vi "Model - DeInit.vi"(8 "error in (no error)":errorcluster, 11 "View Model":T1) -> (0 "error out":errorcluster)   [LabVIEW 2017]
doc: "De-Initialize all View Model Components."
uses:
  Controls/View Model.ctl
  Controls/Shared Model.ctl
  Error Handler/Controls/Error Model.ctl
  Error Handler/Controls/Error Data.ctl
  Error Handler/Controls/Error Type.ctl
  Error Handler/Controls/Error Source.ctl
  Configuration/Controls/Config Model.ctl
  Configuration/Controls/Config CMD.ctl
  Configuration/Controls/Config Command.ctl
  Controller/Controls/Controller Model.ctl
  Controller/Controls/Controller Overhead.ctl
  Controller/Controls/Controller Transaction.ctl
  Controller/Controls/Controller State.ctl
  Configuration/Controls/Config Data Record.ctl
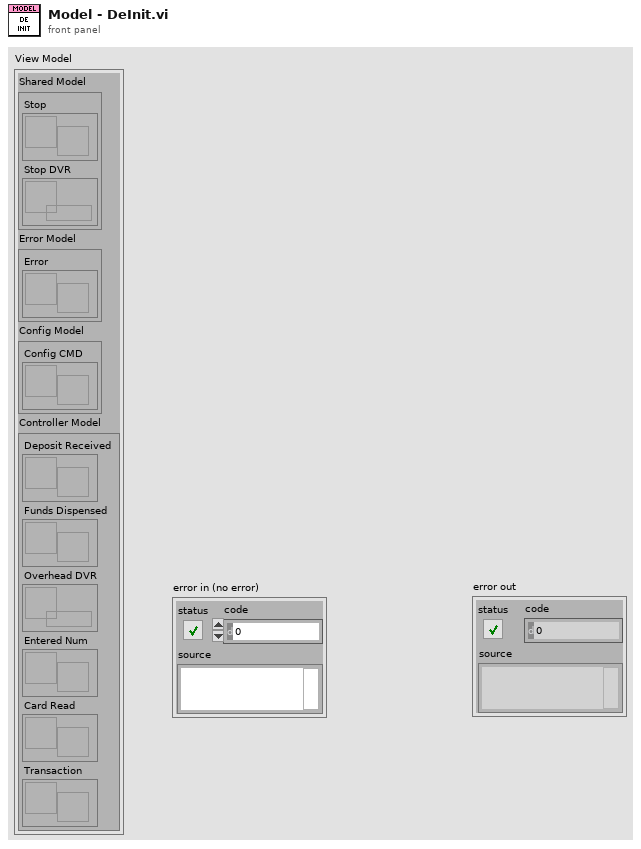
[diagram p1: front panel]
types:
  T1 = typedef "View Model.ctl" = cluster{"Shared Model":T2, "Error Model":T3, "Config Model":T4, "Controller Model":T5}
  T2 = typedef "Shared Model.ctl" = cluster{"Stop":refnum<user-event>, "Stop DVR":refnum<data-value>}
  T3 = typedef "Error Model.ctl" = cluster{"Error":refnum<user-event>}
  T4 = typedef "Config Model.ctl" = cluster{"Config CMD":refnum<user-event>}
  T5 = typedef "Controller Model.ctl" = cluster{"Deposit Received":refnum<user-event>, "Funds Dispensed":refnum<user-event>, "Overhead DVR":refnum<data-value>, "Entered Num":refnum<user-event>, "Card Read":refnum<user-event>, "Transaction":refnum<user-event>}
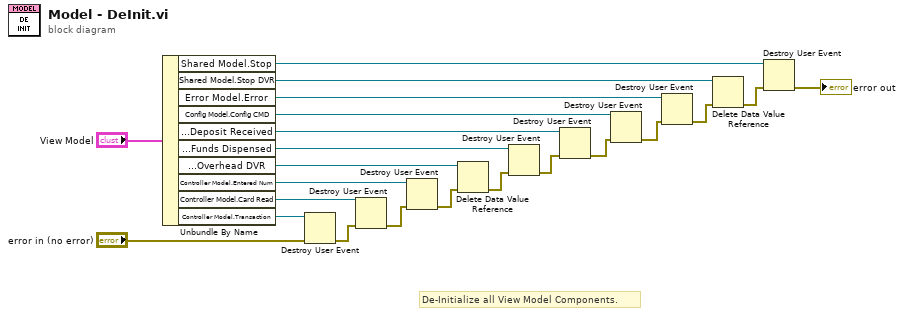
[diagram p0: block diagram]
diagram:
  # "De-Initialize all View Model Components."
  n1 = Unbundle By Name("View Model") -> ("Shared Model.Stop"=w12:refnum<user-event>, "Shared Model.Stop DVR"=w13:refnum<data-value>, "Error Model.Error"=w14:refnum<user-event>, "Config Model.Config CMD"=w15:refnum<user-event>, "Controller Model.Deposit Received"=w16:refnum<user-event>, "Controller Model.Funds Dispensed"=w17:refnum<user-event>, "Controller Model.Overhead DVR"=w18:refnum<data-value>, "Controller Model.Entered Num"=w19:refnum<user-event>, "Controller Model.Card Read"=w20:refnum<user-event>, "Controller Model.Transaction"=w21:refnum<user-event>)
  n2 = Destroy User Event(user event=w21, error in="error in (no error)") -> (error out=w10:errorcluster)
  n3 = Destroy User Event(user event=w20, error in=w10) -> (error out=w9:errorcluster)
  n4 = Destroy User Event(user event=w19, error in=w9) -> (error out=w8:errorcluster)
  n5 = Delete Data Value Reference(data value reference=w18, error in=w8) -> (error out=w7:errorcluster)  [unwired: 1 out]
  n6 = Destroy User Event(user event=w17, error in=w7) -> (error out=w6:errorcluster)
  n7 = Destroy User Event(user event=w16, error in=w6) -> (error out=w5:errorcluster)
  n8 = Destroy User Event(user event=w15, error in=w5) -> (error out=w4:errorcluster)
  n9 = Destroy User Event(user event=w14, error in=w4) -> (error out=w3:errorcluster)
  n10 = Delete Data Value Reference(data value reference=w13, error in=w3) -> (error out=w2:errorcluster)  [unwired: 1 out]
  n11 = Destroy User Event(user event=w12, error in=w2) -> (error out=→"error out":errorcluster)
